vi "Quinn's second method interpolation.vi"(7 "FFT spectrum":dbl[](array[numeric]), 8 "FFT Imm":dbl[](array[numeric]), 11 "FFT real":dbl[](array[numeric])) -> (2 "Index Bin":dbl)   [LabVIEW 2014]
panel:
  out "max index(es)":i32
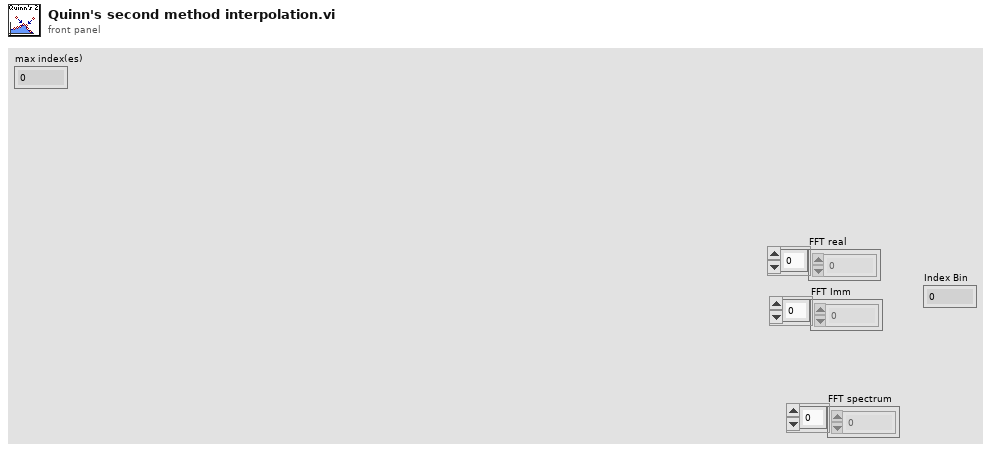
[diagram p1: front panel]
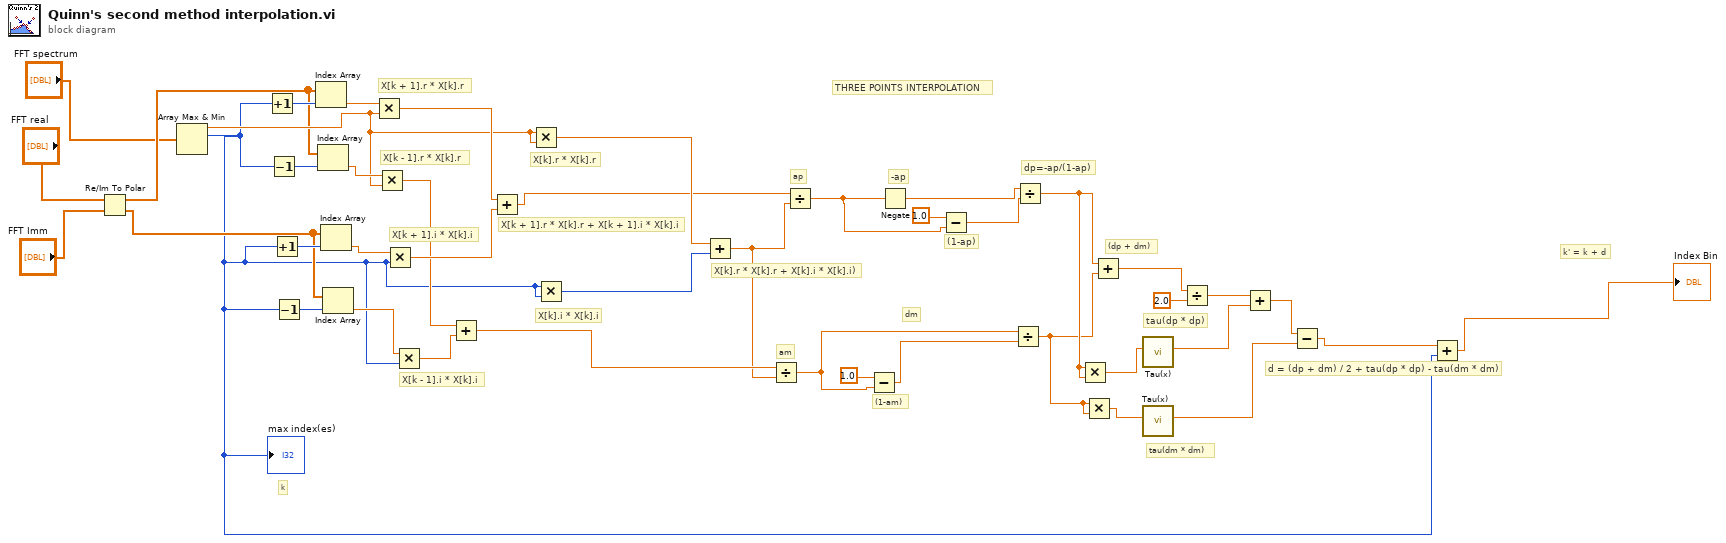
[diagram p0: block diagram]
diagram:
  # "THREE POINTS INTERPOLATION"
  # "k' = k + d"
  # "d = (dp + dm) / 2 + tau(dp * dp) - tau(dm * dm)"
  # "tau(dm * dm)"
  # "tau(dp * dp)"
  # "(dp + dm)"
  # "k"
  # "dm"
  # "(1-am)"
  # "am"
  # "X[k - 1].r * X[k].r"
  # "X[k - 1].i * X[k].i"
  # "dp=-ap/(1-ap)"
  # "(1-ap)"
  # "-ap"
  # "ap"
  # "X[k].r * X[k].r + X[k].i * X[k].i)"
  # "X[k + 1].r * X[k].r + X[k + 1].i * X[k].i"
  # "X[k].r * X[k].r"
  # "X[k].i * X[k].i"
  # "X[k + 1].i * X[k].i"
  # "X[k + 1].r * X[k].r"
  n1 = Re/Im To Polar(2:"FFT Imm", 3:"FFT real") -> (0:w17:dbl[], 1:w18:dbl[])
  n2 = Array Max & Min(array="FFT spectrum") -> (max value=w26:dbl, max index (indices)=w4:i32)  [unwired: 2 out]
  "max index(es)" <- w4
  n3 = Increment(x=w4) -> (x+1=w43:i32)
  n4 = Decrement(x=w4) -> (x-1=w42:i32)
  n5 = Increment(x=w4) -> (x+1=w40:i32)
  n6 = Decrement(x=w4) -> (x-1=w41:i32)
  n7 = Index Array(array=w18, index=w43) -> (element=w39:dbl)
  n8 = Index Array(array=w18, index=w42) -> (element=w27:dbl)
  n9 = Index Array(array=w17, index=w40) -> (element=w38:dbl)
  n10 = Index Array(array=w17, index=w41) -> (element=w28:dbl)
  n11 = Multiply(x=w39, y=w26) -> (x*y=w37:dbl)
  n12 = Multiply(x=w27, y=w26) -> (x*y=w24:dbl)
  n13 = Multiply(x=w38, y=w4) -> (x*y=w36:dbl)
  n14 = Multiply(x=w28, y=w4) -> (x*y=w25:dbl)
  n15 = Add(x=w24, y=w25) -> (x+y=w23:dbl)
  n16 = Add(x=w37, y=w36) -> (x+y=w33:dbl)
  n17 = Multiply(x=w26, y=w26) -> (x*y=w34:dbl)
  n18 = Multiply(x=w4, y=w4) -> (x*y=w35:i32)
  n19 = Add(x=w34, y=w35) -> (x+y=w22:dbl)
  n20 = Divide(x=w23, y=w22) -> (x/y=w20:dbl)
  n21 = Divide(x=w33, y=w22) -> (x/y=w31:dbl)
  n22 = Subtract(x=1.0, y=w20) -> (x-y=w19:dbl)
  n23 = Negate(x=w31) -> (-x=w30:dbl)
  n24 = Subtract(x=1.0, y=w31) -> (x-y=w29:dbl)
  n25 = Divide(x=w20, y=w19) -> (x/y=w7:dbl)
  n26 = Divide(x=w30, y=w29) -> (x/y=w10:dbl)
  n27 = Multiply(x=w10, y=w10) -> (x*y=w11:dbl)
  n28 = Multiply(x=w7, y=w7) -> (x*y=w8:dbl)
  n29 = Add(x=w10, y=w7) -> (x+y=w15:dbl)
  n30 = call "Tau(x).vi"("X"=w11) -> ("Tau"=w12:dbl)  [unwired: 10 in]
  n31 = call "Tau(x).vi"("X"=w8) -> ("Tau"=w6:dbl)  [unwired: 10 in]
  n32 = Divide(x=w15, y=2.0) -> (x/y=w13:dbl)
  n33 = Add(x=w13, y=w12) -> (x+y=w9:dbl)
  n34 = Subtract(x=w9, y=w6) -> (x-y=w5:dbl)
  n35 = Add(x=w5, y=w4) -> (x+y=→"Index Bin":dbl)
